vi "utility.Array To String.vi"(2 "分隔符输入":string, 3 "无符号字节数组":u8[](array[numeric]) format="%02x") -> (0 "字符串数组":string[](array[string]), 1 "命令输出(字符串)":string)   [LabVIEW 2012, in "Lib_UEL.ATE.lvlib" / "Lib_App.lvlib"]
uses:
  Lib_App.lvlib
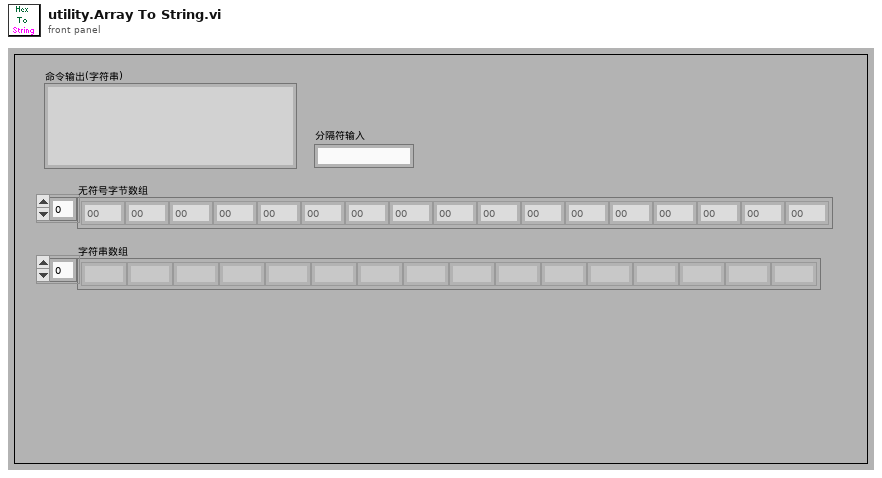
[diagram p1: front panel]
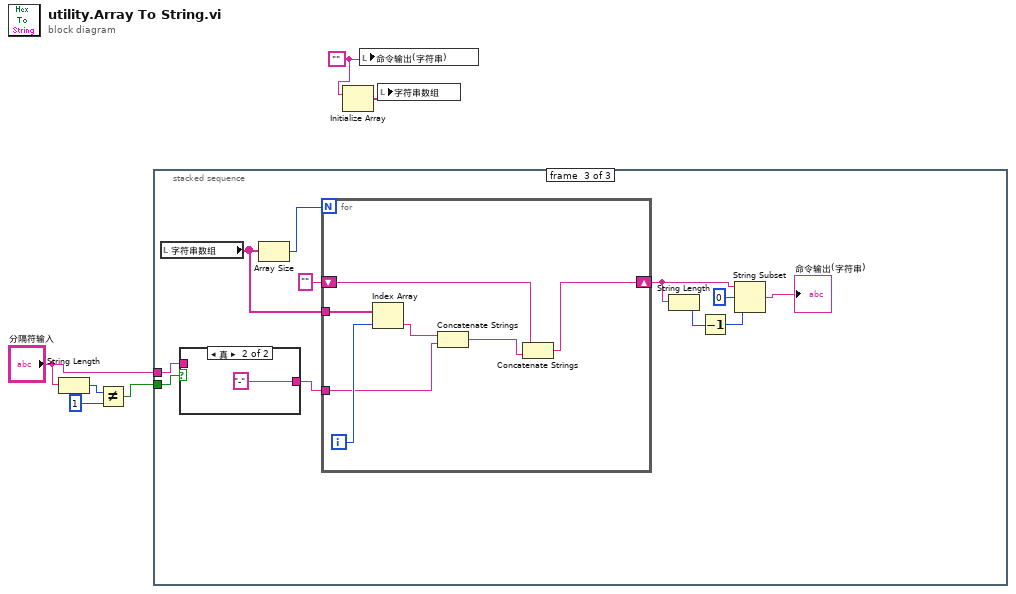
[diagram p0: block diagram]
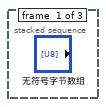
[diagram p2: hidden frame]
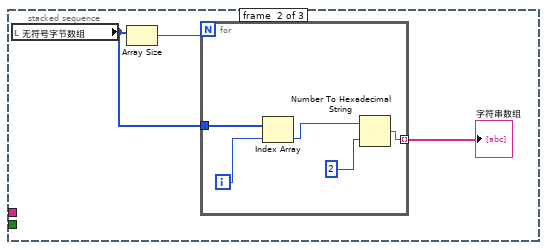
[diagram p3: hidden frame]
diagram:
  w6 = ""
  n1 = String Length(string="分隔符输入") -> (length=w4:i32)
  n2 = Not Equal?(x=w4, y=1) -> (x != y?=w2:bool)
  n3 = stacked-sequence {
    tunnel: w2 -> [_ _ w23]
    tunnel: "分隔符输入" -> [_ _ w21]
    frame #0 {
    }
    frame #1 {
      n4 = local read "无符号字节数组"() -> (w8:u8[])
      n5 = Array Size(array=w8) -> (size(s)=w9:i32)
      n6 = for {
        N: w9 -> [_]
        tunnel: w8 -> [w14]
        tunnel: [w11] -> w7 mode=indexing
        i -> [w13]
        n7 = Index Array(array=w14, index=w13) -> (element=w12:u8)
        n8 = Number To Hexadecimal String(1:2, 2:w12) -> (0:w11:string)
      }
      "字符串数组" <- w7
    }
    frame #2 {
      n9 = local read "字符串数组"() -> (w24:string[])
      n10 = case shown="真" w23 {
        tunnel: [w26 "-" ("字符串")] -> w22
        tunnel: w21 -> [w26 _]
        frame False {
        }
        frame True {
        }
      }
      n11 = Array Size(array=w24) -> (size(s)=w25:i32)
      n12 = for {
        N: w25 -> [_]
        tunnel: w24 -> [w34]
        tunnel: w22 -> [w30]
        shift-right: [w29] -> w17
        shift-left: "" -> [w28]
        i -> [w33]
        n13 = Index Array(array=w34, index=w33) -> (element=w31:string)
        n14 = Concatenate Strings(w31, w30) -> (w32:string)
        n15 = Concatenate Strings(w28, w32) -> (w29:string)
      }
      n16 = String Length(string=w17) -> (length=w16:i32)
      n17 = Decrement(x=w16) -> (x-1=w20:i32)
      n18 = String Subset(string=w17, offset (0)=0 ("偏移量(0)"), length (rest)=w20) -> (substring=→"命令输出(字符串)":string)
    }
  }
  n19 = Initialize Array(w6) -> (w5:string[])  [unwired: 1 in]
  n20 = local write "命令输出(字符串)"(w6) -> ()
  n21 = local write "字符串数组"(w5) -> ()
